vi "Configure Signal - Dual Tone.vi"(7 "output level units":T3, 8 "error in (no error)":errorcluster, 10 "dual tone properties":T1, 11 "Digital Serial in":refnum<class "Digital Serial.lvclass">) -> (0 "error out":errorcluster, 3 "Digital Serial out":refnum<class "Digital Serial.lvclass">)   [LabVIEW 2023, in "Digital Serial.lvclass"]
uses:
  Digital Serial.lvclass
  controls/digital output level units.ctl
  service/generation/controls/dual tone properties.ctl
  service/generation/controls/dual tone types.ctl
  service/generation/controls/sine wave properties.ctl
  Digital Serial.lvclass/Digital Serial.ctl
  <vilib>/PDM Acquisition Toolkit/host/API/Public/Function Generator/Configure Custom Signal (N Ch) - PCM Output Task.vi
  <vilib>/PDM Acquisition Toolkit/host/API/PDM Acquisition Toolkit.lvlib
  service/generation/controls/AudioGenTypeDefs.lvlib
  controls/audio controls.lvlib
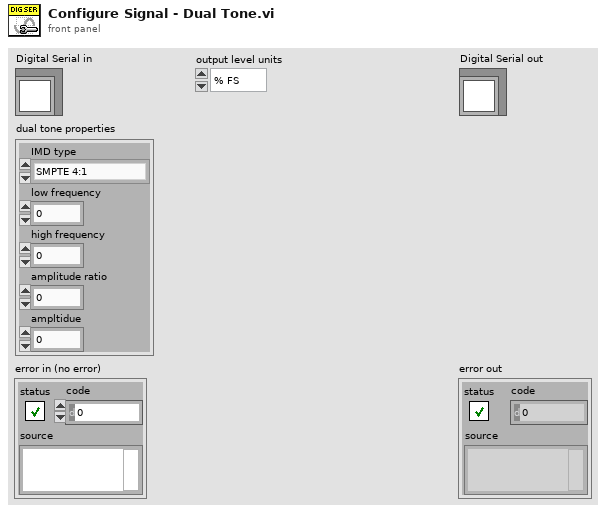
[diagram p1: front panel]
types:
  T1 = typedef "AudioGenTypeDefs.lvlib/dual tone properties.ctl" = cluster{"IMD type":T2, "low frequency":dbl, "high frequency":dbl, "amplitude ratio":dbl, "ampltidue":dbl}
  T2 = typedef "AudioGenTypeDefs.lvlib/dual tone types.ctl" = enum32{"SMPTE 4:1", "DIN", "CCIF 11k-12k", "CCIF 19k-20k", "Custom"}
  T3 = typedef "audio controls.lvlib/digital output level units.ctl" = enum32{"% FS", "dBFS", "V"}
  T4 = typedef "AudioGenTypeDefs.lvlib/sine wave properties.ctl" = cluster{"frequency":dbl, "amplitude":dbl, "phase":dbl}[]
  T5 = typedef "PDM Acquisition Class Library.lvlib/PCM Output Task.lvclass/PCM Output Task DVR.ctl" = refnum<data-value>
  T6 = typedef "PDM Acquisition Class Library.lvlib/I2S Output Task.lvclass/SignalProperties.ctl" = cluster{"cyclic signal":dbl[], "channel parameters":T7[]}
  T7 = typedef "PDM Acquisition Class Library.lvlib/I2S Output Channel.lvclass/GenerationChannelProperties.ctl" = cluster{"cyclic period":dbl, "cyclic phase offset":dbl, "gain":dbl}
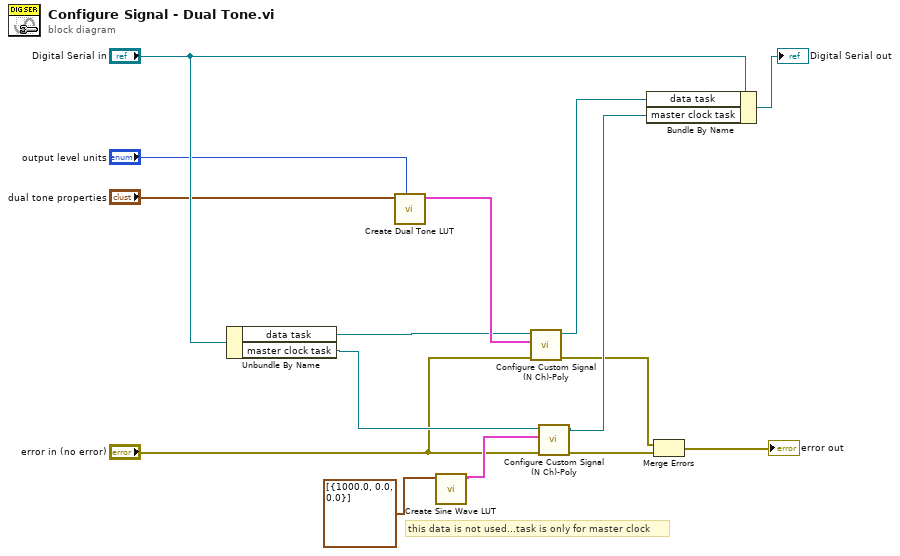
[diagram p0: block diagram]
diagram:
  # "this data is not used...task is only for master clock"
  n1 = Unbundle By Name("Digital Serial in") -> ("data task"=w12:T5, "master clock task"=w11:T5)
  n2 = call "Create Dual Tone LUT.vi"("output level units"="output level units", "dual tone properties"="dual tone properties") -> ("Signal Properties"=w15:T6)  [unwired: 9 in]
  n3 = call "Create Sine Wave LUT.vi"("sine wave properties"=T4 [{"frequency"=1000.0, "amplitude"=0.0, "phase"=0.0}]) -> ("Signal Properties"=w14:T6)  [unwired: 10 in]
  n4 = call-poly <vilib>:"Configure Custom Signal (N Ch)-Poly.vi"("error in"="error in (no error)", "signal parameters"=w15, "PCM output task in"=w12) -> ("error out"=w6:errorcluster, "PCM output task out"=w8:T5)  [unwired: 7 in]
  n5 = call-poly <vilib>:"Configure Custom Signal (N Ch)-Poly.vi"("error in"="error in (no error)", "signal parameters"=w14, "PCM output task in"=w11) -> ("error out"=w5:errorcluster, "PCM output task out"=w7:T5)  [unwired: 7 in]
  n6 = Bundle By Name(cluster="Digital Serial in", "data task"=w8, "master clock task"=w7) -> (→"Digital Serial out":refnum<class "Digital Serial.lvclass">)
  n7 = Merge Errors(w6, w5) -> (→"error out":errorcluster)
